vi "saveSetup.vi"(4 "error in (no error)":errorcluster, 6 "Configuration":T2) -> (0 "error out":errorcluster, 1 "Canceled?":bool, 2 "Configuration Written":T1 {"Select Mode:" items=["Custom", "Imaging", "300 All", "600 UV", "600 Blue", "600 Mid", "600 Red", "1200 m0", "1200 m1", "1200 m2", "1200 m3", "1200 m4", "1200 m5", "1200 m6", "1200 m7", "1200 RESOLVE", "400 m1", "400 m2", "930 m1", "930 m2", "930 m3", "930 m4", "930 m5", "930 m6", "400KL"]})   [LabVIEW 2015]
uses:
  GUI/GSP_GUI_global.vi
  GSCS Scripting/Utils/GSP_ObsConfig.llb/configuration.ctl
panel:
  in  "Save to":path
  out "?":string
  in  "Save":bool
  in  "Configuration Name":string="default"
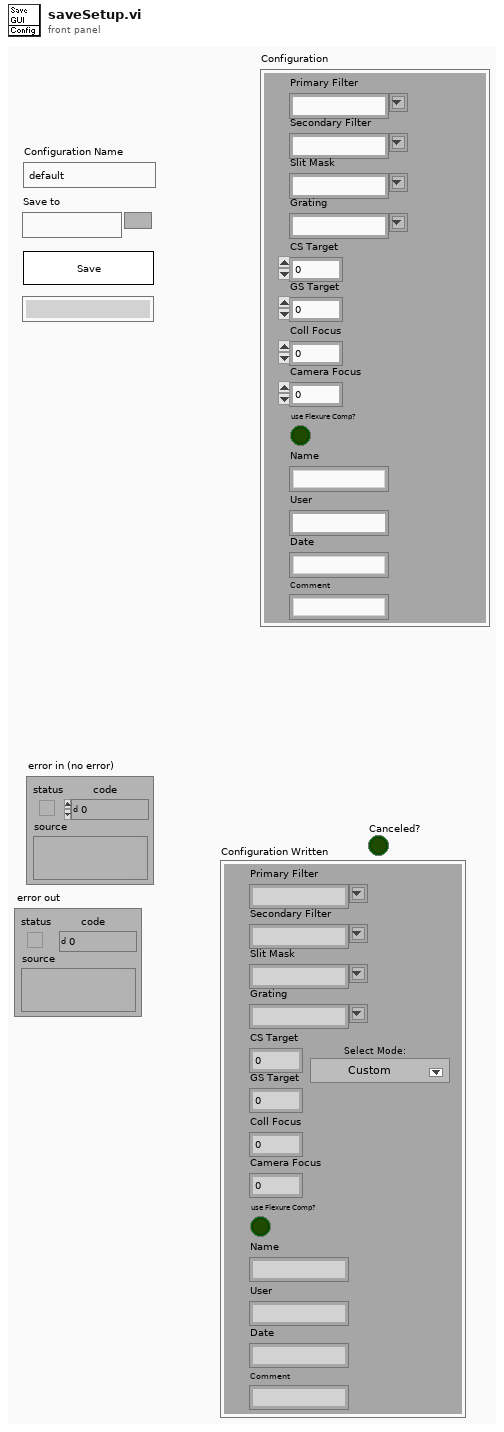
[diagram p1: front panel]
types:
  T1 = typedef "configuration.ctl" = cluster{"Primary Filter":string, "Secondary Filter":string, "Slit Mask":string, "Grating":string, "CS Target":dbl, "GS Target":dbl, "Coll Focus":i32, "Camera Focus":i32, "Name":string, "User":string, "Date":string, "Comment":string, "use Flexure Comp?":bool, "Select Mode:":u16}
  T2 = cluster{"Primary Filter":string, "Secondary Filter":string, "Slit Mask":string, "Grating":string, "CS Target":dbl, "GS Target":dbl, "Coll Focus":i32, "Camera Focus":i32, "Name":string, "User":string, "Date":string, "Comment":string, "use Flexure Comp?":bool}
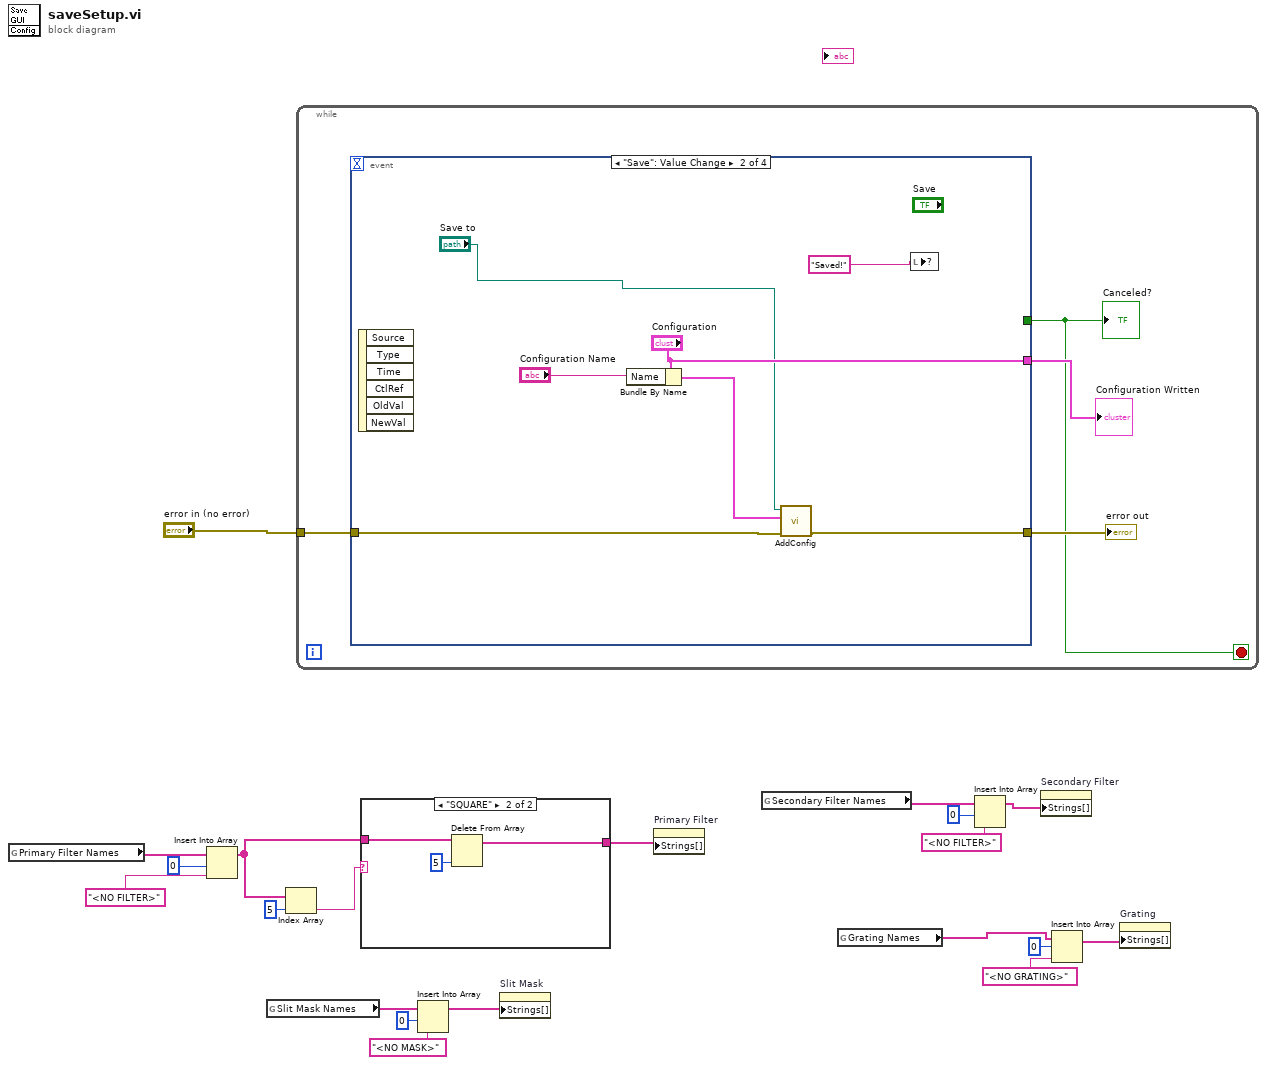
[diagram p0: block diagram]
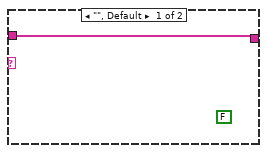
[diagram p2: hidden frame]
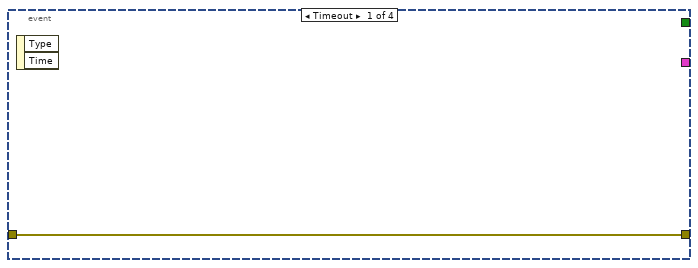
[diagram p3: hidden frame]
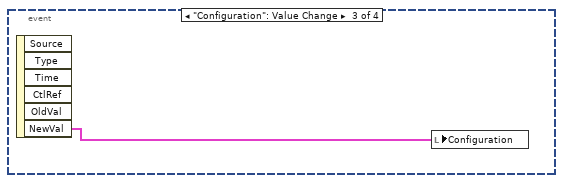
[diagram p4: hidden frame]
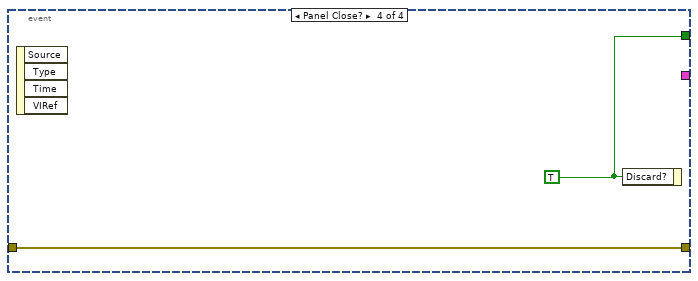
[diagram p5: hidden frame]
diagram:
  n1 = global read "GSP_GUI_global.vi" "Primary Filter Names"() -> (w18:string[])
  n2 = Insert Into Array(array=w18, index=0, new element="<NO FILTER>" ("new element/subarray")) -> (w16:string[])
  n3 = global read "GSP_GUI_global.vi" "Slit Mask Names"() -> (w7:string[])
  n4 = Index Array(array=w16, index=5) -> (element=w14:string)
  n5 = while {
    tunnel: "error in (no error)" -> [w24]
    stop <- w21 stop-if-true
    n6 = event shown="[1] \"Save\": Value Change" {
      selector: _ -> [_ _ _ _]
      dyn-events: _ -> [_ _ _ _]
      timeout: _ -> [_ _ _ _]
      tunnel: [_ _ _ w34] -> w21
      tunnel: w24 -> [w25 w31 _ w35]
      tunnel: [w25 w30 _ w35] -> w23
      tunnel: [_ "Configuration" _ _] -> w22
      event Timeout {
        n7 = event-data() -> ()  [unwired: 1 in, 2 out]
      }
      event "Save": Value Change {
        n8 = event-data() -> ()  [unwired: 1 in, 6 out]
        n9 = Bundle By Name(cluster="Configuration", "Name"="Configuration Name") -> (w29:T2)
        n10 = call "AddConfig.vi"("error in (no error)"=w31, "Configuration In"=w29, "path"="Save to") -> ("error out"=w30:errorcluster)  [unwired: 4 in]
        n11 = local write item#7("Saved!") -> ()
      }
      event "Configuration": Value Change {
        n12 = event-data() -> ("NewVal"=w33:T2)  [unwired: 1 in, 5 out]
        n13 = local write "Configuration"(w33) -> ()
      }
      event Panel Close? {
        w34 = TRUE
        n14 = event-data() -> ()  [unwired: 1 in, 4 out]
        n15 = event-data("Discard?"=w34) -> ()  [unwired: 1 in, 1 out]
      }
    }
    "error out" <- w23
    "Canceled?" <- w21
    "Configuration Written" <- w22
  }
  n16 = case shown="\"SQUARE\"" w14 {
    tunnel: w16 -> [w36 w39]
    tunnel: [w36 w37] -> w2
    frame "", Default {
      (unwired) FALSE ("5 hole or 6 hole wheel?")
    }
    frame "SQUARE" {
      n17 = Delete From Array(array=w39, index=5) -> (array with subset deleted=w37:string[])  [unwired: 1 in, 1 out]
    }
  }
  n18 = Insert Into Array(array=w7, index=0, new element="<NO MASK>" ("new element/subarray")) -> (w1:string[])
  n19 = property on="Slit Mask" class="CmbBox"("Strings[]"=w1) -> ()  [unwired: 2 in, 2 out]
  n20 = property on="Primary Filter" class="CmbBox"("Strings[]"=w2) -> ()  [unwired: 2 in, 2 out]
  n21 = global read "GSP_GUI_global.vi" "Secondary Filter Names"() -> (w11:string[])
  n22 = global read "GSP_GUI_global.vi" "Grating Names"() -> (w8:string[])
  n23 = Insert Into Array(array=w11, index=0, new element="<NO FILTER>" ("new element/subarray")) -> (w3:string[])
  n24 = property on="Secondary Filter" class="CmbBox"("Strings[]"=w3) -> ()  [unwired: 2 in, 2 out]
  n25 = Insert Into Array(array=w8, index=0, new element="<NO GRATING>" ("new element/subarray")) -> (w4:string[])
  n26 = property on="Grating" class="CmbBox"("Strings[]"=w4) -> ()  [unwired: 2 in, 2 out]
